vi "Set Buffer.vi"(6 "Set? (Ignored)":bool=TRUE, 7 "Config in":refnum<class "Carya Config.lvclass">, 8 "error in (no error)":errorcluster, 11 "Carya Config (Buffer) in":refnum<class "CConfig Nonpersistant Buffer.lvclass">) -> (0 "error out":errorcluster, 2 "Replace?":bool=TRUE, 3 "Carya Config (Buffer) out":refnum<class "CConfig Nonpersistant Buffer.lvclass">)   [LabVIEW 2013, in "CConfig Nonpersistant Buffer.lvclass"]
doc: "Copyright 2018, Carya Automatisering, Wiebe Walstra."
uses:
  CConfig Nonpersistant Buffer.lvclass
  Carya Config.lvclass
  CConfig Nonpersistant Buffer.lvclass/CConfig Nonpersistant Buffer.ctl
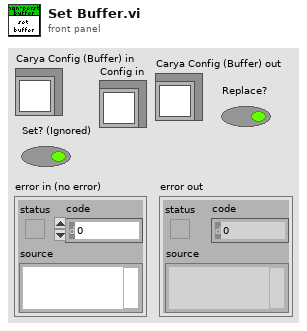
[diagram p1: front panel]
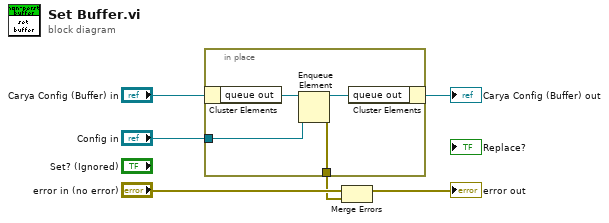
[diagram p0: block diagram]
diagram:
  n1 = in-place {
    in-place-border: [w8] -> w2
    in-place-border: "Config in" -> [w7]
    n2 = in-place-cluster #1("Carya Config (Buffer) in") -> ("queue out"=w10:refnum<queue>)
    n3 = Enqueue Element(queue=w10, element=w7) -> (queue out=w9:refnum<queue>, error out=w8:errorcluster)  [unwired: 2 in, 1 out]
    n4 = in-place-cluster #1("queue out"=w9) -> (→"Carya Config (Buffer) out":refnum<class "CConfig Nonpersistant Buffer.lvclass">)
  }
  n5 = Merge Errors("error in (no error)", w2) -> (→"error out":errorcluster)
